vi "CalcPosArray.vi"(8 "Inbetween diff":dbl=3.0, 9 "Min diff":dbl=0.5, 10 "Posit Array":T1[](array[typedef]), 11 "All Lines":T2) -> (1 "Modified?":bool, 3 "All Lines out":T2, 5 "Selected array":i32[](array[numeric]))   [LabVIEW 2014]
uses:
  Libraries/Map Data Folder/All-Lines.ctl
  Libraries/Map Data Folder/LineCluster.ctl
  Libraries/Map Data Folder/LineConnection.ctl
  Libraries/Contact Data/Position.ctl
  Libraries/Map Data Folder/Map Data.lvlib
  Libraries/Contact Data/Contact Data.lvlib
panel:
  in  "Max multi":dbl=2.0
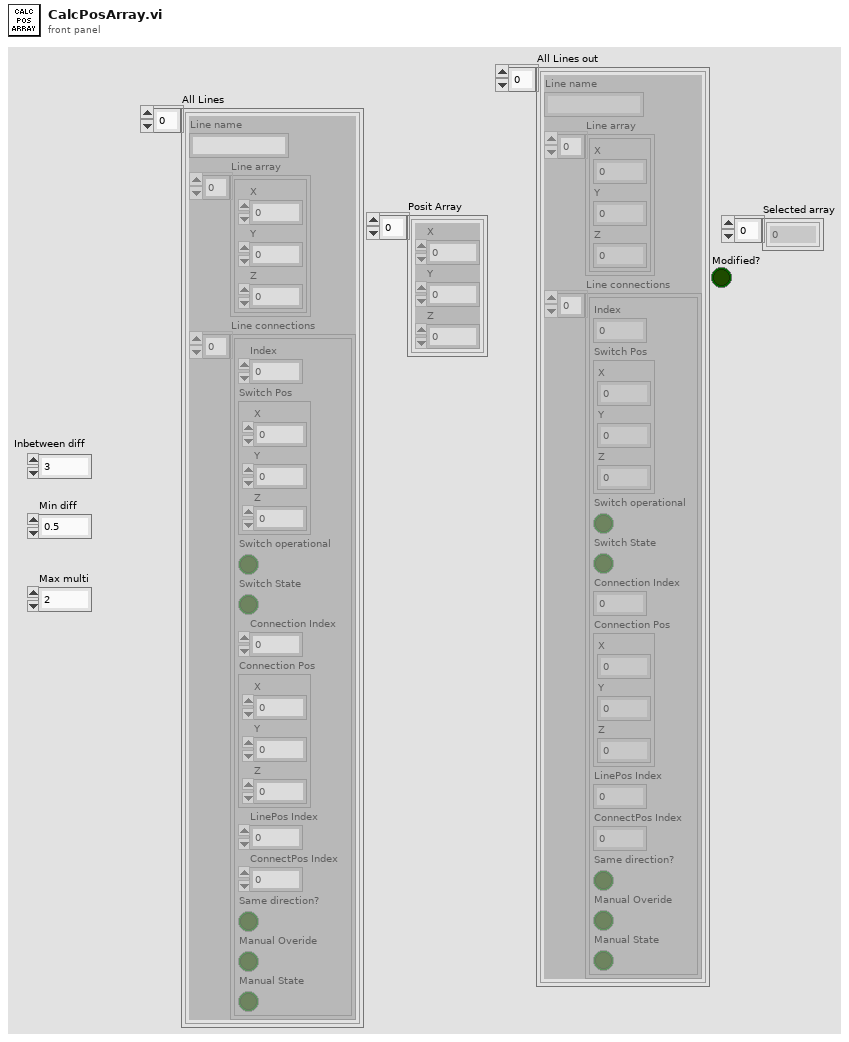
[diagram p1: front panel]
types:
  T1 = typedef "Contact Data.lvlib/Position.ctl" = cluster{"X":dbl, "Y":dbl, "Z":dbl}
  T2 = typedef "Map Data.lvlib/All-Lines.ctl" = T3[]
  T3 = typedef "Map Data.lvlib/LineCluster.ctl" = cluster{"Line name":string, "Line array":cluster{"X":dbl, "Y":dbl, "Z":dbl}[], "Line connections":T4[]}
  T4 = typedef "LineConnection.ctl" = cluster{"Index":i32, "Switch Pos":cluster{"X":dbl, "Y":dbl, "Z":dbl}, "Switch operational":bool, "Switch State":bool, "Connection Index":i32, "Connection Pos":cluster{"X":dbl, "Y":dbl, "Z":dbl}, "LinePos Index":i32, "ConnectPos Index":i32, "Same direction?":bool, "Manual Overide":bool, "Manual State":bool}
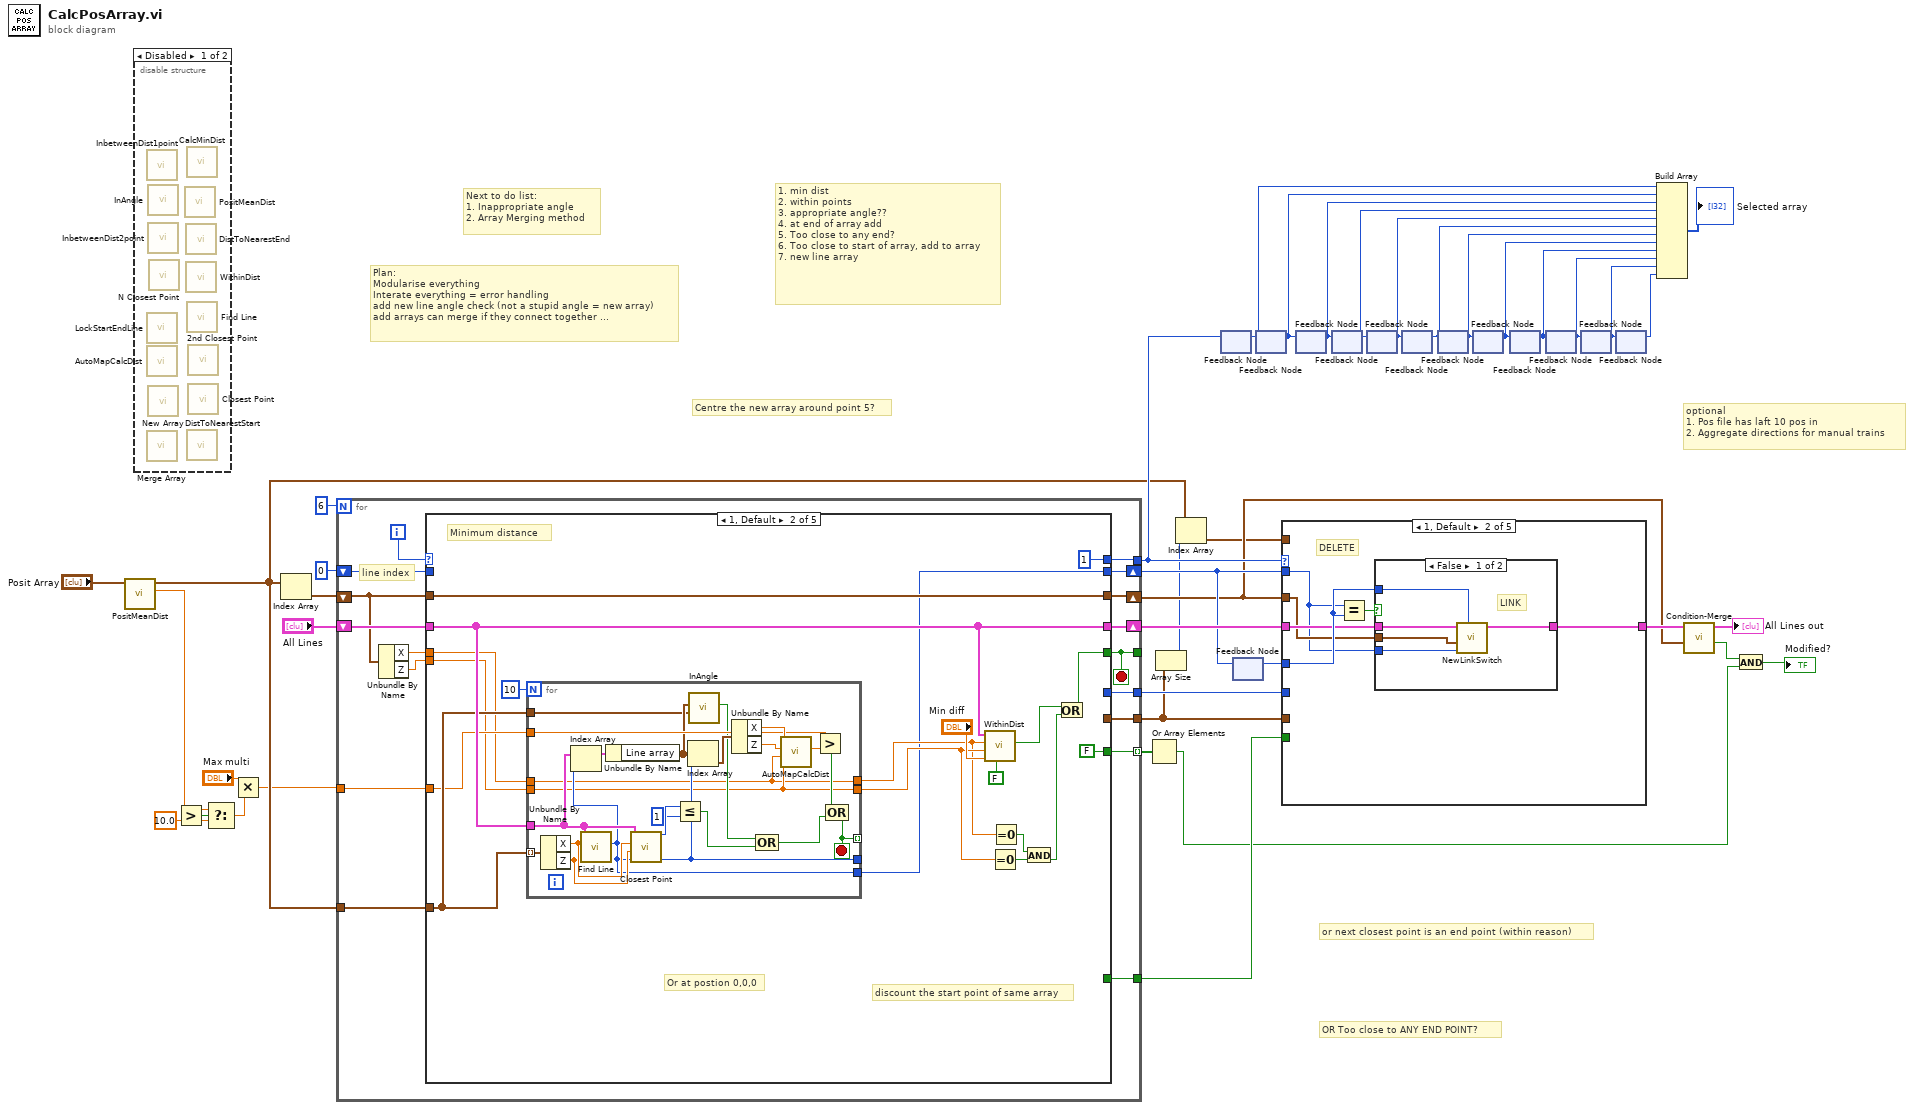
[diagram p0: block diagram]
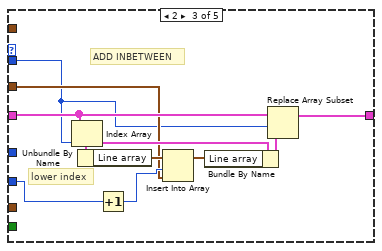
[diagram p5: hidden frame]
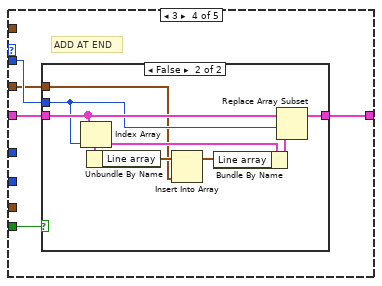
[diagram p6: hidden frame]
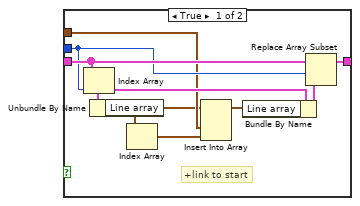
[diagram p7: hidden frame]
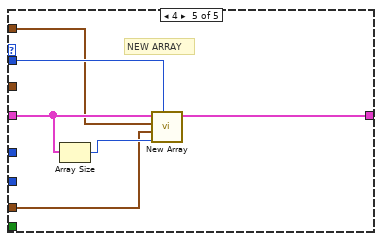
[diagram p8: hidden frame]
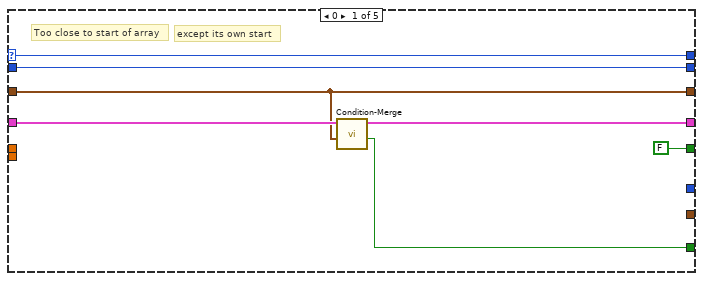
[diagram p9: hidden frame]
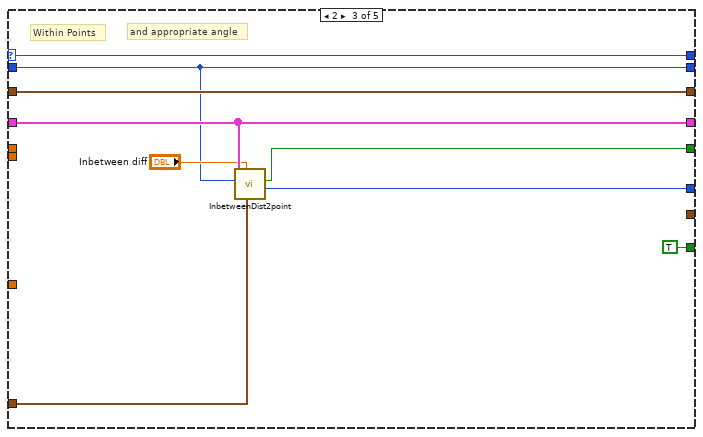
[diagram p10: hidden frame]
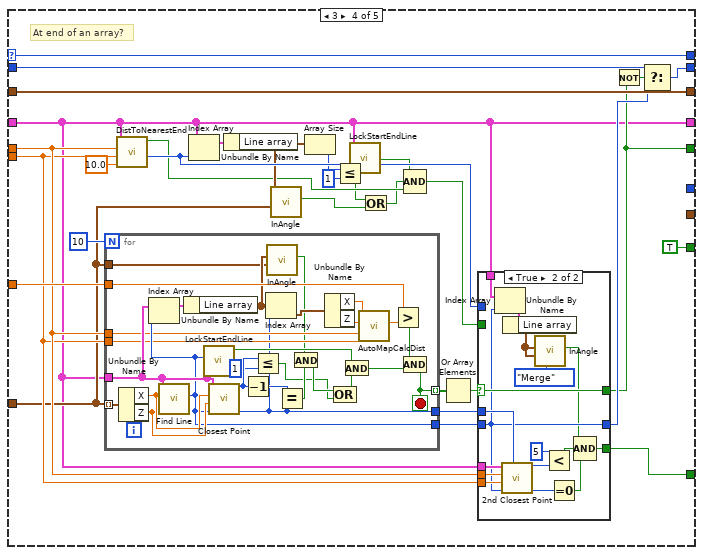
[diagram p11: hidden frame]
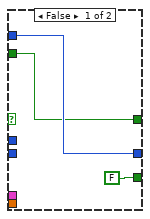
[diagram p12: hidden frame]
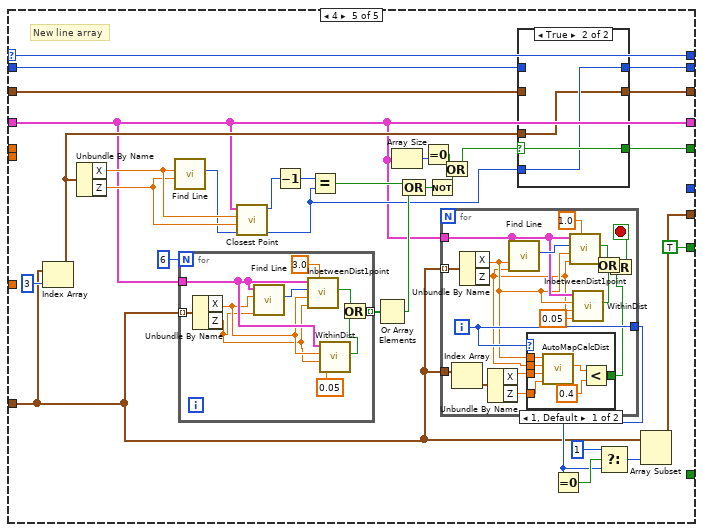
[diagram p13: hidden frame]
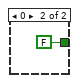
[diagram p14: hidden frame]
diagram:
  w9 = 10.0 ("y")
  # "Centre the new array around point 5?"
  # "or next closest point is an end point (within reason)"
  # "OR Too close to ANY END POINT?"
  # "Next to do list:\n1. Inappropriate angle\n2. Array Merging method"
  # "optional \n1. Pos file has laft 10 pos in\n2. Aggregate directions for manual trains"
  # "1. min dist\n2. within points\n3. appropriate angle??\n4. at end of array add \n5. Too close to any end?\n6. Too close to start of array, add to array\n7. new line array"
  # "Plan:\nModularise everything\nInterate everything = error handling\nadd new line angle check (not a stupid angle = new array)\nadd arrays can merge if they connect together ..."
  n1 = call "PositMeanDist.vi"("Posit Array"="Posit Array") -> ("Latest dist"=w5:dbl, "Posit Array"=w11:T1[])  [unwired: 7 in, 2 out]
  n2 = disable-structure shown="Disabled" {
    frame Disabled {
      n3 = call "InbetweenDist1point.vi"() -> ()  [unwired: 9 in, 3 out]
      n4 = call "LockStartEndLine.vi"() -> ()  [unwired: 11 in, 1 out]
      n5 = call "AutoMapCalcDist.vi"() -> ()  [unwired: 11 in, 1 out]
      n6 = call "Merge Array.vi"() -> ()  [unwired: 11 in, 1 out]
      n7 = call "InAngle.vi"() -> ()  [unwired: 11 in, 1 out]
      n8 = call "InbetweenDist2point.vi"() -> ()  [unwired: 9 in, 3 out]
      n9 = call "New Array.vi"() -> ()  [unwired: 11 in, 1 out]
      n10 = call "N Closest Point.vi"() -> ()  [unwired: 10 in, 2 out]
      n11 = call "PositMeanDist.vi"() -> ()  [unwired: 8 in, 4 out]
      n12 = call "DistToNearestEnd.vi"() -> ()  [unwired: 9 in, 3 out]
      n13 = call "WithinDist.vi"() -> ()  [unwired: 10 in, 2 out]
      n14 = call "CalcMinDist.vi"() -> ()  [unwired: 10 in, 2 out]
      n15 = call "Find Line.vi"() -> ()  [unwired: 8 in, 4 out]
      n16 = call "DistToNearestStart.vi"() -> ()  [unwired: 9 in, 3 out]
      n17 = call "2nd Closest Point.vi"() -> ()  [unwired: 10 in, 2 out]
      n18 = call "Closest Point.vi"() -> ()  [unwired: 9 in, 3 out]
    }
    frame Enabled {
    }
  }
  n19 = Greater?(x=w5, y=w9) -> (0:w10:bool)
  n20 = Select(t=w5, s=w10, f=w9) -> (s? t:f=w7:dbl)
  n21 = Multiply(x="Max multi", y=w7) -> (x*y=w6:dbl)
  n22 = Index Array(array=w11) -> (element=w24:T1)  [unwired: 1 in]
  n23 = for {
    N: 6 -> [_]
    shift-right: [w56] -> w38
    shift-left: "All Lines" -> [w57]
    tunnel: [w55] -> w34
    tunnel: [w54] -> _
    shift-right: [w53] -> w36
    shift-left: 0 ("Nearest Line") -> [w52]
    tunnel: [w51] -> w37
    shift-right: [w47] -> w25
    shift-left: w24 -> [w48]
    tunnel: w11 -> [w46]
    tunnel: [w45] -> w16
    tunnel: [w44] -> w13
    tunnel: w6 -> [w43]
    tunnel: [w42] -> w4 mode=indexing
    i -> [w58]
    stop <- w54 stop-if-true
    # "line index"
    n24 = Unbundle By Name(w48) -> ("X"=w50:dbl, "Z"=w49:dbl)
    n25 = case shown="1, Default" w58 {
      selector: w58 -> [w65 _ w116 w147 w226]
      tunnel: w57 -> [w62 w75 w115 w125 w201]
      tunnel: [w61 w75 w115 w125 w201] -> w56
      tunnel: w50 -> [_ w70 _ w136 _]
      tunnel: w49 -> [_ w71 _ w135 _]
      tunnel: [w65 1 w116 w147 w226] -> w55
      tunnel: [FALSE ("In range?") w82 w110 w130 w215] -> w54
      tunnel: [w63 w67 w111 w143 w211] -> w53
      tunnel: w52 -> [w63 _ w111 w138 w212]
      tunnel: [_ _ w113 _ _] -> w51
      tunnel: [w60 w80 w112 w146 w213] -> w47
      tunnel: w48 -> [w60 w80 w112 w146 w214]
      tunnel: w46 -> [_ w74 w109 w133 w197]
      tunnel: [_ _ _ _ w207] -> w45
      tunnel: [_ _ _ w141 _] -> w44
      tunnel: w43 -> [_ w72 _ w139 _]
      tunnel: [w59 FALSE ("Modified?") TRUE ("Modified?") TRUE ("Modified?") TRUE ("Modified?")] -> w42
      frame 0 {
        # "except its own start"
        # "Too close to start of array"
        n26 = call "Condition-Merge.vi"("Input Pos"=w60, "All Lines"=w62) -> ("Modified?"=w59:bool, "array out"=w61:T2)  [unwired: 8 in]
      }
      frame 1, Default {
        # "discount the start point of same array"
        # "Or at postion 0,0,0"
        # "Minimum distance"
        n27 = for {
          N: 10 -> [_]
          tunnel: w74 -> [w107] mode=indexing
          tunnel: w75 -> [w99]
          tunnel: [w92] -> _ mode=indexing
          tunnel: [w98] -> w67
          tunnel: w70 -> [w85]
          tunnel: w71 -> [w86]
          tunnel: [w96] -> _
          tunnel: w72 -> [w97]
          tunnel: w74 -> [w94]
          tunnel: [w86] -> w69
          tunnel: [w85] -> w68
          stop <- w92 stop-if-true
          n28 = Unbundle By Name(w107) -> ("X"=w106:dbl, "Z"=w105:dbl)
          n29 = call "Find Line.vi"("Z"=w105, "X"=w106, "All Lines"=w99) -> ("Nearest Line"=w98:i32)  [unwired: 5 in, 3 out]
          n30 = Index Array(array=w99, index=w98) -> (element=w104:T3)
          n31 = Unbundle By Name(w104) -> ("Line array"=w95:cluster{"X":dbl, "Y":dbl, "Z":dbl}[])
          n32 = call "Closest Point.vi"("index"=w98, "Y in"=w105, "X in"=w106, "All Lines"=w99) -> ("Index on Line"=w96:i32, "Array size"=w91:i32)  [unwired: 5 in, 1 out]
          n33 = Less Or Equal?(x=w91, y=1) -> (x <= y?=w89:bool)
          n34 = Index Array(array=w95, index=w96) -> (element=w103:cluster{"X":dbl, "Y":dbl, "Z":dbl})
          n35 = call "InAngle.vi"("2nd Array (Start)"=w94, "Base Array (End)"=w95) -> ("In Angle?"=w88:bool)  [unwired: 9 in]
          n36 = Unbundle By Name(w103) -> ("X"=w102:dbl, "Z"=w101:dbl)
          n37 = Compound Arithmetic op=OR(w88, w89) -> (w87:bool)
          n38 = call "AutoMapCalcDist.vi"("Y2"=w86, "X2"=w85, "Y1"=w101, "X1"=w102) -> ("Distance"=w100:dbl)  [unwired: 7 in]
          n39 = Greater?(x=w97, y=w100) -> (0:w93:bool)
          n40 = Compound Arithmetic op=OR(w93, w87) -> (w92:bool)
        }
        n41 = call "WithinDist.vi"("Discount start?"=FALSE, "Range"="Min diff", "Z"=w69, "X"=w68, "All Lines"=w75) -> ("In Range?"=w83:bool)  [unwired: 5 in, 1 out]
        n42 = Equal To 0?(x=w69) -> (x = 0?=w81:bool)
        n43 = Equal To 0?(x=w68) -> (x = 0?=w77:bool)
        n44 = And(x=w77, y=w81) -> (x .and. y?=w78:bool)
        n45 = Or(x=w83, y=w78) -> (x .or. y?=w82:bool)
      }
      frame 2 {
        # "and appropriate angle"
        # "Within Points"
        n46 = call "InbetweenDist2point.vi"("Posit Array"=w109, "Inbetween diff"="Inbetween diff", "Index"=w111, "All Lines"=w115) -> ("Lower index"=w113:i32, "In range?"=w110:bool)  [unwired: 5 in, 1 out]
      }
      frame 3 {
        # "At end of an array?"
        n47 = for {
          N: 10 -> [_]
          tunnel: w133 -> [w195] mode=indexing
          tunnel: w125 -> [w185]
          tunnel: [w175] -> w145 mode=indexing
          tunnel: [w184] -> w137
          tunnel: w136 -> [w181]
          tunnel: w135 -> [w182]
          tunnel: [w180] -> w140
          tunnel: w139 -> [w183]
          tunnel: w133 -> [w178]
          stop <- w175 stop-if-true
          n48 = Unbundle By Name(w195) -> ("X"=w193:dbl, "Z"=w192:dbl)
          n49 = call "Find Line.vi"("Z"=w192, "X"=w193, "All Lines"=w185) -> ("Nearest Line"=w184:i32)  [unwired: 5 in, 3 out]
          n50 = Index Array(array=w185, index=w184) -> (element=w190:T3)
          n51 = Unbundle By Name(w190) -> ("Line array"=w179:cluster{"X":dbl, "Y":dbl, "Z":dbl}[])
          n52 = call "LockStartEndLine.vi"("index"=w184, "All Lines"=w185) -> ("Not Locked?"=w191:bool)  [unwired: 9 in]
          n53 = call "Closest Point.vi"("index"=w184, "Y in"=w192, "X in"=w193, "All Lines"=w185) -> ("Index on Line"=w180:i32, "Array size"=w171:i32)  [unwired: 5 in, 1 out]
          n54 = Decrement(x=w171) -> (x-1=w194:i32)
          n55 = Less Or Equal?(x=w171, y=1) -> (x <= y?=w168:bool)
          n56 = Index Array(array=w179, index=w180) -> (element=w189:cluster{"X":dbl, "Y":dbl, "Z":dbl})
          n57 = call "InAngle.vi"("2nd Array (Start)"=w178, "Base Array (End)"=w179) -> ("In Angle?"=w172:bool)  [unwired: 9 in]
          n58 = Equal?(x=w194, y=w180) -> (x = y?=w169:bool)
          n59 = And(x=w172, y=w169) -> (x .and. y?=w173:bool)
          n60 = Unbundle By Name(w189) -> ("X"=w188:dbl, "Z"=w187:dbl)
          n61 = Compound Arithmetic op=OR(w173, w168) -> (w174:bool)
          n62 = And(x=w191, y=w174) -> (x .and. y?=w176:bool)
          n63 = call "AutoMapCalcDist.vi"("Y2"=w182, "X2"=w181, "Y1"=w187, "X1"=w188) -> ("Distance"=w186:dbl)  [unwired: 7 in]
          n64 = Greater?(x=w183, y=w186) -> (0:w177:bool)
          n65 = Compound Arithmetic op=AND(w177, w176) -> (w175:bool)
        }
        n66 = call "DistToNearestEnd.vi"("Any End"=10.0, "Z"=w135, "X"=w136, "All Lines 2"=w125) -> ("Index"=w127:i32, "In range?"=w123:bool)  [unwired: 5 in, 1 out]
        n67 = Index Array(array=w125, index=w127) -> (element=w132:T3)
        n68 = Unbundle By Name(w132) -> ("Line array"=w124:cluster{"X":dbl, "Y":dbl, "Z":dbl}[])
        n69 = call "InAngle.vi"("2nd Array (Start)"=w133, "Base Array (End)"=w124) -> ("In Angle?"=w122:bool)  [unwired: 9 in]
        n70 = Array Size(array=w124) -> (size(s)=w120:i32)
        n71 = Less Or Equal?(x=w120, y=1) -> (x <= y?=w118:bool)
        n72 = call "LockStartEndLine.vi"("index"=w127, "All Lines"=w125) -> ("Not Locked?"=w126:bool)  [unwired: 9 in]
        n73 = Or(x=w118, y=w122) -> (x .or. y?=w121:bool)
        n74 = Compound Arithmetic op=AND(w126, w121, w123) -> (w128:bool)
        n75 = Or Array Elements(Boolean array=w145) -> (logical OR=w129:bool)
        n76 = case shown="True" w129 {
          selector: w129 -> [_ w161]
          tunnel: [FALSE w154] -> w141
          tunnel: w140 -> [_ w159]
          tunnel: w137 -> [_ w158]
          tunnel: w136 -> [_ w164]
          tunnel: w135 -> [_ w163]
          tunnel: w125 -> [_ w162]
          tunnel: [w150 w158] -> w131
          tunnel: [w149 w161] -> w130
          tunnel: w128 -> [w149 _]
          tunnel: w127 -> [w150 _]
          tunnel: w125 -> [_ w157]
          frame False {
          }
          frame True {
            n77 = Index Array(array=w157, index=w158) -> (element=w160:T3)
            n78 = call "2nd Closest Point.vi"("index to ignore"=w159, "line index"=w158, "Y in"=w163, "X in"=w164, "All Lines"=w162) -> ("Index on Line"=w165:i32, "Array size"=w167:i32)  [unwired: 5 in]
            n79 = Unbundle By Name(w160) -> ("Line array"=w156:cluster{"X":dbl, "Y":dbl, "Z":dbl}[])
            n80 = call "InAngle.vi"("Function"=enum16{"Posit", "Merge"}."Merge", "2nd Array (Start)"=w156, "Base Array (End)"=w156) -> ("In Angle?"=w151:bool)  [unwired: 8 in]
            n81 = Less?(x=5, y=w167) -> (x < y?=w152:bool)
            n82 = Equal To 0?(x=w165) -> (x = 0?=w153:bool)
            n83 = Compound Arithmetic op=AND(w151, w152, w153) -> (w154:bool)
          }
        }
        n84 = Not(x=w130) -> (.not. x?=w144:bool)
        n85 = Select(t=w138, s=w144, f=w131) -> (s? t:f=w143:i32)
      }
      frame 4 {
        # "New line array"
        n86 = Index Array(array=w197, index=3) -> (element=w209:T1)
        n87 = Unbundle By Name(w209) -> ("X"=w219:dbl, "Z"=w218:dbl)
        n88 = call "Find Line.vi"("Z"=w218, "X"=w219) -> ("Nearest Line"=w217:i32)  [unwired: 6 in, 3 out]
        n89 = for {
          N: 6 -> [_]
          tunnel: w197 -> [w267] mode=indexing
          tunnel: w201 -> [w263]
          tunnel: [w262] -> w198 mode=indexing
          n90 = Unbundle By Name(w267) -> ("X"=w259:dbl, "Z"=w258:dbl)
          n91 = call "Find Line.vi"("Z"=w258, "X"=w259, "All Lines"=w263) -> ("Nearest Line"=w266:i32)  [unwired: 5 in, 3 out]
          n92 = call "InbetweenDist1point.vi"("Inbetween diff"=3.0, "Z"=w258, "X"=w259, "Index"=w266, "All Lines"=w263) -> ("In range?"=w261:bool)  [unwired: 4 in, 2 out]
          n93 = call "WithinDist.vi"("Range"=0.05, "Z"=w258, "X"=w259, "All Lines"=w263) -> ("In Range?"=w260:bool)  [unwired: 6 in, 1 out]
          n94 = Or(x=w261, y=w260) -> (x .or. y?=w262:bool)
        }
        n95 = call "Closest Point.vi"("index"=w217, "Y in"=w218, "X in"=w219, "All Lines"=w201) -> ("Index on Line"=w210:i32, "Array size"=w222:i32)  [unwired: 5 in, 1 out]
        n96 = Decrement(x=w222) -> (x-1=w225:i32)
        n97 = Equal?(x=w225, y=w210) -> (x = y?=w224:bool)
        n98 = Or Array Elements(Boolean array=w198) -> (logical OR=w221:bool)
        n99 = Array Size(array=w201) -> (size(s)=w200:i32)
        n100 = Compound Arithmetic op=OR(w224, w221) -> (w223:bool)
        n101 = Equal To 0?(x=w200) -> (x = 0?=w199:bool)
        n102 = Not(x=w223) -> (.not. x?=w216:bool)
        n103 = for {
          tunnel: w201 -> [w238]
          tunnel: w197 -> [w241] mode=indexing
          tunnel: [w235] -> w205
          tunnel: w197 -> [w234]
          i -> [w235]
          stop <- w228 stop-if-true
          n104 = Index Array(array=w234) -> (element=w233:T1)  [unwired: 1 in]
          n105 = Unbundle By Name(w241) -> ("X"=w232:dbl, "Z"=w231:dbl)
          n106 = Unbundle By Name(w233) -> ("X"=w230:dbl, "Z"=w229:dbl)
          n107 = call "Find Line.vi"("Z"=w231, "X"=w232, "All Lines"=w238) -> ("Nearest Line"=w243:i32)  [unwired: 5 in, 3 out]
          n108 = case shown="1, Default" w235 {
            tunnel: w232 -> [w250 _]
            tunnel: w231 -> [w249 _]
            tunnel: w230 -> [w248 _]
            tunnel: w229 -> [w247 _]
            tunnel: [w245 FALSE] -> w227
            frame 1, Default {
              n109 = call "AutoMapCalcDist.vi"("Y2"=w247, "X2"=w248, "Y1"=w249, "X1"=w250) -> ("Distance"=w246:dbl)  [unwired: 7 in]
              n110 = Less?(x=w246, y=0.4) -> (x < y?=w245:bool)
            }
            frame 0 {
            }
          }
          n111 = call "InbetweenDist1point.vi"("Inbetween diff"=1.0, "Z"=w231, "X"=w232, "Index"=w243, "All Lines"=w238) -> ("In range?"=w240:bool)  [unwired: 4 in, 2 out]
          n112 = call "WithinDist.vi"("Range"=0.05, "Z"=w231, "X"=w232, "All Lines"=w238) -> ("In Range?"=w236:bool)  [unwired: 6 in, 1 out]
          n113 = Or(x=w240, y=w236) -> (x .or. y?=w237:bool)
          n114 = Or(x=w237, y=w227) -> (x .or. y?=w228:bool)
        }
        n115 = Or(x=w199, y=w216) -> (x .or. y?=w202:bool)
        n116 = case shown="True" w202 {
          selector: w202 -> [w252 w257]
          tunnel: [w252 w257] -> w215
          tunnel: w214 -> [w253 _]
          tunnel: [w253 w255] -> w213
          tunnel: w212 -> [w254 _]
          tunnel: [w254 w256] -> w211
          tunnel: w210 -> [_ w256]
          tunnel: w209 -> [_ w255]
          frame False {
          }
          frame True {
          }
        }
        n117 = Equal To 0?(x=w205) -> (x = 0?=w206:bool)
        n118 = Select(t=1, s=w206, f=w205) -> (s? t:f=w203:i32)
        n119 = Array Subset(array=w197, length=w203) -> (w207:T1[])  [unwired: 1 in]
      }
    }
  }
  n120 = Or Array Elements(Boolean array=w4) -> (logical OR=w2:bool)
  n121 = Array Size(array=w16) -> (size(s)=w15:i32)
  n122 = Index Array(array=w11, index=w15) -> (element=w14:T1)
  n123 = feedback #1() -> (w33:i32)  [unwired: 1 in]
  n124 = feedback-in #1(w34) -> ()
  n125 = feedback #2() -> (w35:i32)  [unwired: 1 in]
  n126 = feedback-in #2(w36) -> ()
  n127 = feedback #3() -> (w32:i32)  [unwired: 1 in]
  n128 = feedback-in #3(w33) -> ()
  n129 = case shown="1, Default" w34 {
    tunnel: w38 -> [w268 w272 w284 w294 w317]
    tunnel: [w268 w271 w285 w295 w318] -> w27
    tunnel: w37 -> [_ _ w282 _ _]
    tunnel: w25 -> [_ w270 w283 w292 _]
    tunnel: w36 -> [_ w269 w281 w293 w315]
    tunnel: w14 -> [_ _ _ _ w313]
    tunnel: w35 -> [_ w273 _ _ _]
    tunnel: w16 -> [_ _ _ _ w314]
    tunnel: w13 -> [_ _ _ w291 _]
    frame 0 {
      # "MERGE"
    }
    frame 1, Default {
      # "DELETE"
      n130 = Equal?(x=w269, y=w273) -> (x = y?=w274:bool)
      n131 = case shown="False" w274 {
        tunnel: w273 -> [w278 _]
        tunnel: w270 -> [w279 _]
        tunnel: w269 -> [w277 _]
        tunnel: w272 -> [w276 w280]
        tunnel: [w275 w280] -> w271
        frame False {
          # "LINK"
          n132 = call "NewLinkSwitch.vi"("prev index"=w278, "new index"=w277, "new element"=w279, "array"=w276) -> ("array out"=w275:T2)  [unwired: 7 in]
        }
        frame True {
        }
      }
    }
    frame 2 {
      # "ADD INBETWEEN"
      # "lower index"
      n133 = Index Array(array=w284, index=w281) -> (element=w289:T3)
      n134 = Unbundle By Name(w289) -> ("Line array"=w288:cluster{"X":dbl, "Y":dbl, "Z":dbl}[])
      n135 = Increment(x=w282) -> (x+1=w286:i32)
      n136 = Insert Into Array(array=w288, index=w286, new element=w283) -> (w287:cluster{"X":dbl, "Y":dbl, "Z":dbl}[])
      n137 = Bundle By Name(cluster=w289, "Line array"=w287) -> (w290:T3)
      n138 = Replace Array Subset(array=w284, new element=w290, index=w281) -> (w285:T2)
    }
    frame 3 {
      # "ADD AT END"
      n139 = case shown="False" w291 {
        tunnel: [w301 w308] -> w295
        tunnel: w294 -> [w300 w307]
        tunnel: w293 -> [w299 w306]
        tunnel: w292 -> [w298 w305]
        frame True {
          # "+link to start"
          n140 = Index Array(array=w300, index=w299) -> (element=w303:T3)
          n141 = Unbundle By Name(w303) -> ("Line array"=w297:cluster{"X":dbl, "Y":dbl, "Z":dbl}[])
          n142 = Index Array(array=w297) -> (element=w296:cluster{"X":dbl, "Y":dbl, "Z":dbl})  [unwired: 1 in]
          n143 = Insert Into Array(array=w297, new element #1=w298, new element #2=w296) -> (w302:cluster{"X":dbl, "Y":dbl, "Z":dbl}[])  [unwired: 1 in]
          n144 = Bundle By Name(cluster=w303, "Line array"=w302) -> (w304:T3)
          n145 = Replace Array Subset(array=w300, new element=w304, index=w299) -> (w301:T2)
        }
        frame False {
          n146 = Index Array(array=w307, index=w306) -> (element=w311:T3)
          n147 = Unbundle By Name(w311) -> ("Line array"=w310:cluster{"X":dbl, "Y":dbl, "Z":dbl}[])
          n148 = Insert Into Array(array=w310, new element=w305) -> (w309:cluster{"X":dbl, "Y":dbl, "Z":dbl}[])  [unwired: 1 in]
          n149 = Bundle By Name(cluster=w311, "Line array"=w309) -> (w312:T3)
          n150 = Replace Array Subset(array=w307, new element=w312, index=w306) -> (w308:T2)
        }
      }
    }
    frame 4 {
      # "NEW ARRAY"
      n151 = Array Size(array=w317) -> (size(s)=w316:i32)
      n152 = call "New Array.vi"("prev index"=w315, "new index"=w316, "Array"=w314, "prev element"=w313, "array"=w317) -> ("array out"=w318:T2)  [unwired: 6 in]
    }
  }
  n153 = feedback #4() -> (w31:i32)  [unwired: 1 in]
  n154 = feedback-in #4(w32) -> ()
  n155 = feedback #5() -> (w30:i32)  [unwired: 1 in]
  n156 = feedback-in #5(w31) -> ()
  n157 = feedback #6() -> (w29:i32)  [unwired: 1 in]
  n158 = feedback-in #6(w30) -> ()
  n159 = feedback #7() -> (w23:i32)  [unwired: 1 in]
  n160 = feedback-in #7(w29) -> ()
  n161 = feedback #8() -> (w22:i32)  [unwired: 1 in]
  n162 = feedback-in #8(w23) -> ()
  n163 = feedback #9() -> (w21:i32)  [unwired: 1 in]
  n164 = feedback-in #9(w22) -> ()
  n165 = feedback #10() -> (w20:i32)  [unwired: 1 in]
  n166 = feedback-in #10(w21) -> ()
  n167 = feedback #11() -> (w19:i32)  [unwired: 1 in]
  n168 = feedback-in #11(w20) -> ()
  n169 = feedback #12() -> (w18:i32)  [unwired: 1 in]
  n170 = feedback-in #12(w19) -> ()
  n171 = feedback #13() -> (w17:i32)  [unwired: 1 in]
  n172 = feedback-in #13(w18) -> ()
  n173 = Build Array(w33, w32, w31, w30, w29, w23, w22, w21, w20, w19, w18, w17) -> (→"Selected array":i32[])
  n174 = call "Condition-Merge.vi"("Input Pos"=w25, "All Lines"=w27) -> ("Modified?"=w3:bool, "array out"=→"All Lines out":T2)  [unwired: 8 in]
  n175 = And(x=w3, y=w2) -> (x .and. y?=→"Modified?":bool)
